vi "RemoveAnyWhitespaceFromString.vi"(11 "String in":string) -> (3 "String out":string)   [LabVIEW 2020]
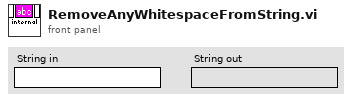
[diagram p1: front panel]
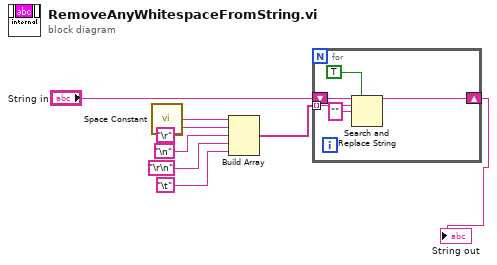
[diagram p0: block diagram]
diagram:
  n1 = call "Space Constant.vi"() -> ("String"=w2:string)
  n2 = Build Array(w2, "\r", "\n", "\r\n", "\t") -> (w7:string[])
  n3 = for {
    tunnel: w7 -> [w12] mode=indexing
    shift-right: [w10] -> w8
    shift-left: "String in" -> [w13]
    n4 = Search and Replace String(replace all?=TRUE ("replace all? (F)"), input string=w13, search string=w12, replace string="" ("replace string (\"\")")) -> (result string=w10:string)  [unwired: 4 in, 3 out]
  }
  "String out" <- w8
